vi "GetPowerSpectrum.vi"(11 "Fft Results (in)":csg[](array[numeric])) -> (3 "PowerSpectrum (out)":sgl[](array[numeric]))   [LabVIEW 2015, in "SETI_LV.lvlib"]
uses:
  SETI_LV.lvlib
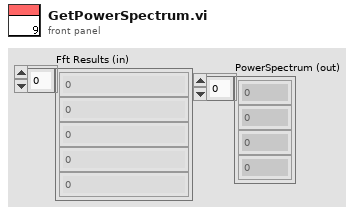
[diagram p1: front panel]
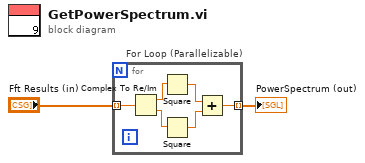
[diagram p0: block diagram]
diagram:
  n1 = for "For Loop (Parallelizable)" {
    tunnel: "Fft Results (in)" -> [w8] mode=indexing
    tunnel: [w5] -> w1 mode=indexing
    n2 = Complex To Re/Im(x + iy=w8) -> (x=w7:sgl, y=w6:sgl)
    n3 = Square(x=w7) -> (x^2=w4:sgl)
    n4 = Square(x=w6) -> (x^2=w3:sgl)
    n5 = Add(x=w4, y=w3) -> (x+y=w5:sgl)
  }
  "PowerSpectrum (out)" <- w1
